vi "Main_NIAI.vi"(8 "error in":errorcluster) -> (0 "error out":errorcluster)   [LabVIEW 2019]
uses:
  _ctrl/create-rw-close.ctl
  cnt_NIAI.ctl
  SubVIs/common/_ctrl/system-status.ctl
  _ctrl/init-r-stop.ctl
  SubVIs/common/Glob_Ref.vi
  Durability/common/Global 1.vi
panel:
  out "n":i32
  out "data":waveform(dbl)[](graph)
  out "n":i32
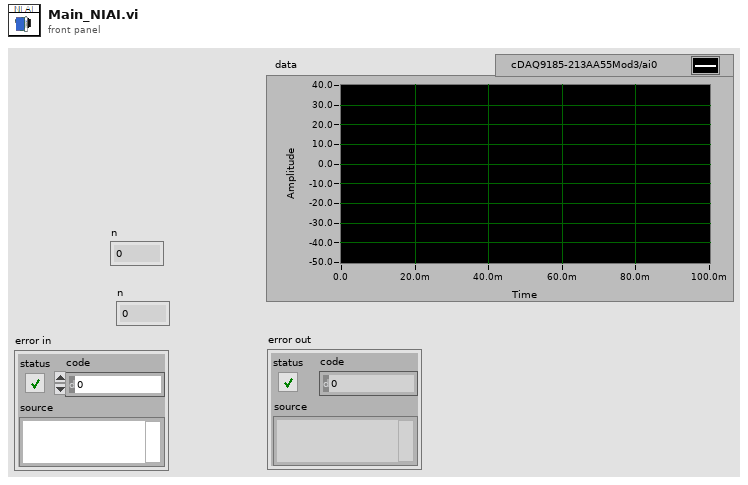
[diagram p1: front panel]
types:
  T1 = typedef "create-rw-close.ctl" = enum16{"create", "write", "read", "delete", "close"}
  T2 = typedef "cnt_NIAI.ctl" = enum16{"Open", "Read", "Close"}
  T3 = typedef "init-r-stop.ctl" = enum16{"ini", "read", "stop"}
  T4 = typedef "system-status.ctl" = enum16{"Initial", "Update", "Clear", "Read"}
  T5 = typedef "start.ctl" = enum16{"init", "open", "set", "start", "stop", "read", "read_items", "query", "close", "T_single", "reset", "exit"}
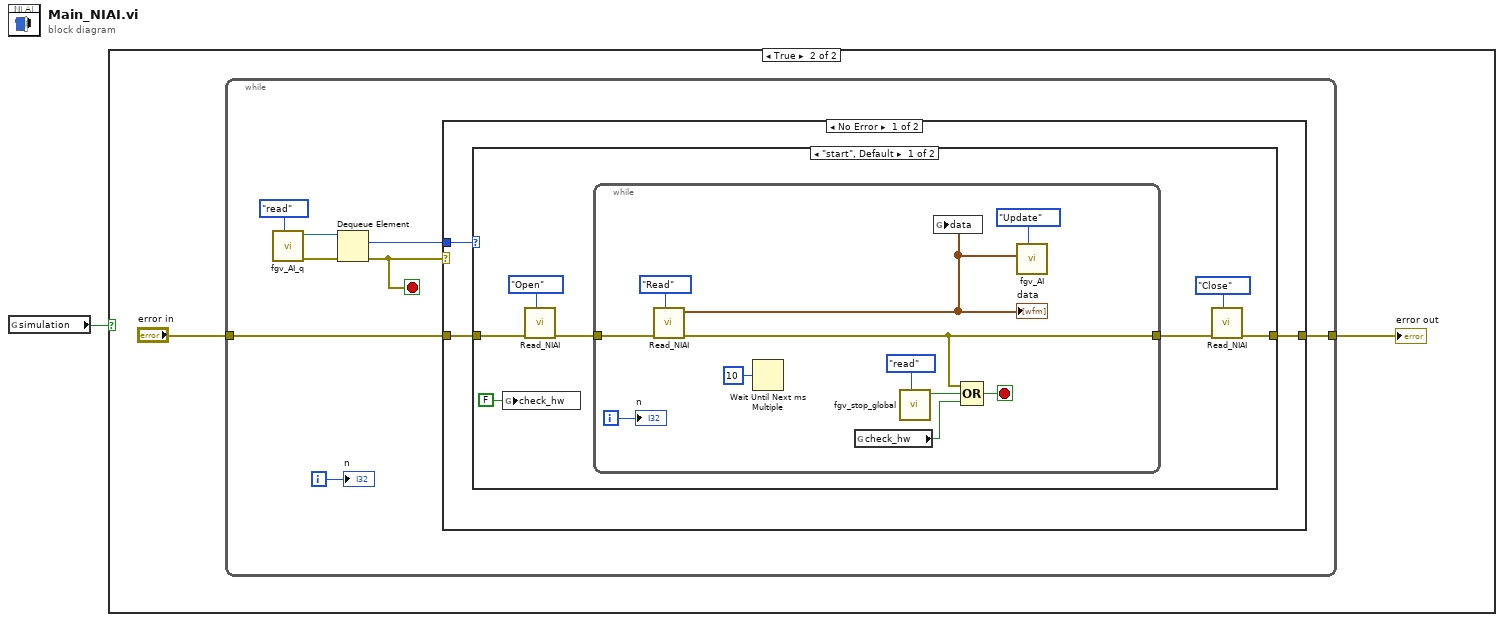
[diagram p0: block diagram]
diagram:
  n1 = global read "Glob_Ref.vi" "simulation"() -> (w1:bool)
  n2 = case shown="True" w1 {
    frame False {
    }
    frame True {
      n3 = while {
        tunnel: "error in" -> [w5]
        tunnel: [w4] -> w2
        i -> [w9]
        stop <- w10 stop-if-true
        n4 = call "fgv_AI_q.vi"("cmd"=create-rw-close."read") -> ("error out"=w6:errorcluster, "queue out"=w7:refnum<queue>)  [unwired: 9 in]
        n5 = Dequeue Element(queue=w7, error in (no error)=w6) -> (element=w11:T5, error out=w10:errorcluster)  [unwired: 1 in, 2 out]
        n6 = case shown="No Error" w10 {
          tunnel: w11 -> [w14 _]
          tunnel: w5 -> [w13 w34]
          tunnel: [w12 w34] -> w4
          frame No Error {
            n7 = case shown="\"start\", Default" w14 {
              tunnel: w13 -> [w16 w33]
              tunnel: [w15 w33] -> w12
              frame "start", Default {
                n8 = global write "Glob_Ref.vi" "check_hw"(FALSE ("check_hw")) -> ()
                n9 = call "Read_NIAI.vi"("cnt"=cnt_NIAI."Open", "error in"=w16) -> ("error out"=w20:errorcluster)  [unwired: 7 in, 2 out]
                n10 = while {
                  tunnel: w20 -> [w31]
                  tunnel: [w28] -> w18
                  i -> [w26]
                  stop <- w27 stop-if-true
                  n11 = call "Read_NIAI.vi"("cnt"=cnt_NIAI."Read", "error in"=w31) -> ("error out"=w28:errorcluster, "data"=w29:waveform(dbl)[])  [unwired: 7 in, 1 out]
                  "data" <- w29
                  n12 = Wait Until Next ms Multiple(millisecond multiple=u32 10) -> ()  [unwired: 1 out]
                  n13 = global read "Glob_Ref.vi" "check_hw"() -> (w22:bool)
                  n14 = call "fgv_stop_global.vi"("cmd"=init-r-stop."read") -> ("stop"=w23:bool)  [unwired: 10 in]
                  n15 = global write "Global 1.vi" "data"(w29) -> ()
                  n16 = Compound Arithmetic op=OR(w28, w23, w22) -> (w27:bool)
                  n17 = call "fgv_AI.vi"("Mode"=system-status."Update", "Value"=w29) -> ()  [unwired: 7 in, 3 out]
                  "n" <- w26
                }
                n18 = call "Read_NIAI.vi"("cnt"=cnt_NIAI."Close", "error in"=w18) -> ("error out"=w15:errorcluster)  [unwired: 7 in, 2 out]
              }
              frame "stop" {
              }
            }
          }
          frame Error {
          }
        }
        "n" <- w9
      }
      "error out" <- w2
    }
  }
